vi "AI test.vi"() -> ()   [LabVIEW 2017]
panel:
  in  "Reade":bool
  in  "stop":bool
  out "AI  Init  array":errorcluster[](array[cluster])
  out "Analog error":bool
  out "Analog Fault Counts":i32[](array[numeric])
  out "AI Data 0":waveform(dbl)[](graph)
  out "AI Data 1":waveform(dbl)[](graph)
  out "AI Data 2":waveform(dbl)[](graph)
  out "AI Error":errorcluster[](array[cluster])
  out "AI loop time":dbl format="%.6g"
  out "AI data 2":waveform(dbl)[](array[waveform])
  out "AI data 1":waveform(dbl)[](array[waveform])
  out "AI data 0":waveform(dbl)[](array[waveform])
  in  "RATE (Hz)":dbl=5000.0
  out "physical channels 2":string="DemoDevice,BID#0/ai0:1" caption="property value"
  out "physical channels 1":string="DemoDevice,BID#0/ai0:1" caption="property value"
  out "physical channels 0":string="DemoDevice,BID#0/ai0:1" caption="property value"
  out "AI Task2":u32
  out "AI Task1":u32
  out "AI Task0":u64
  in  "SAMPLES":dbl=500.0
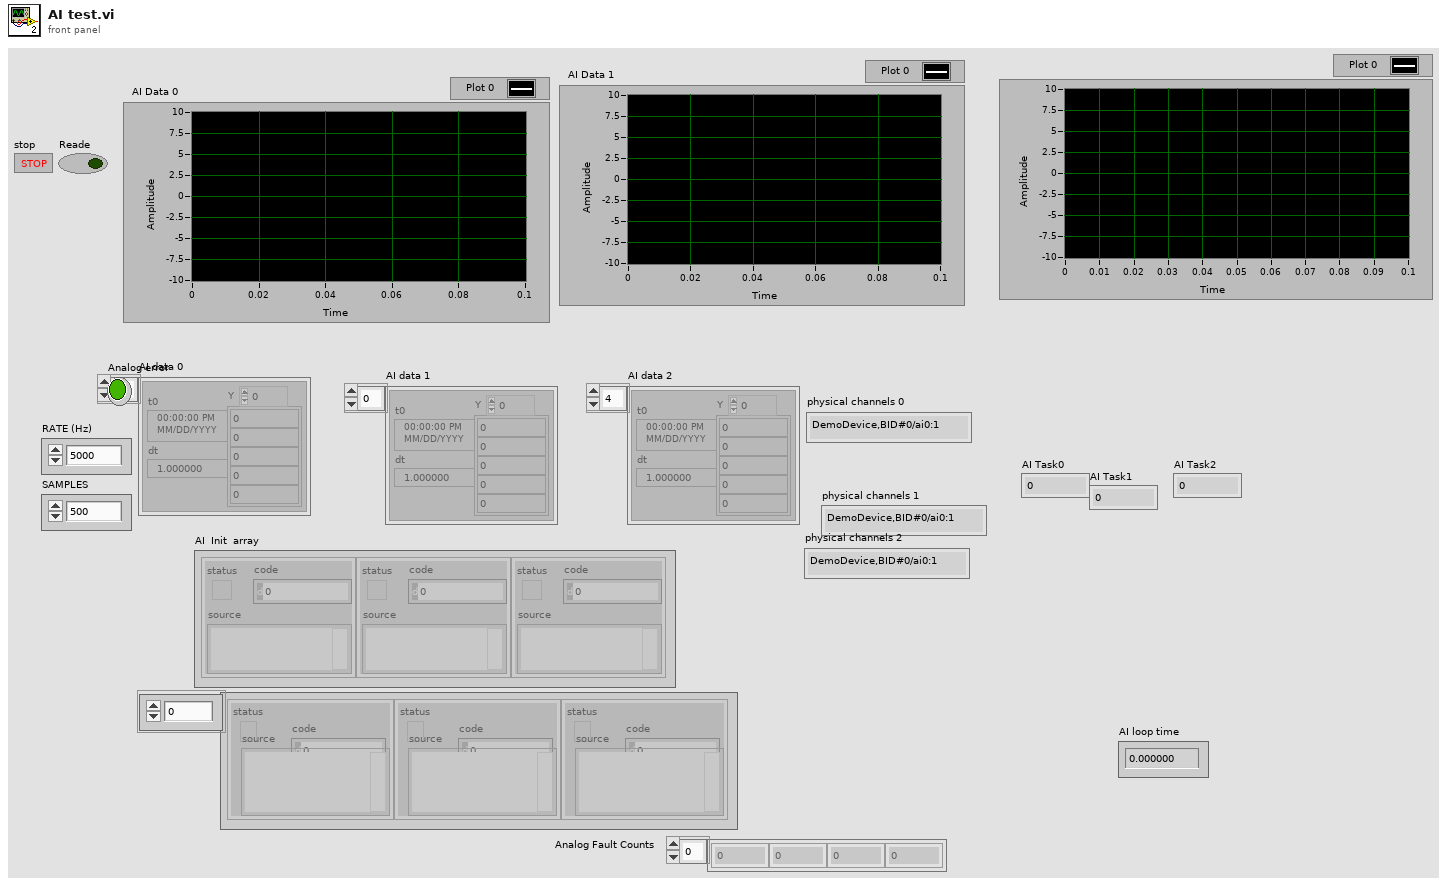
[diagram p1: front panel]
types:
  T1 = cluster{"OUT SERVER ADDRESS":string, "FROM ACCOUNT":string, "USER NAME":string, "PASSWORD":string, "TEST MAIL":bool, "TEST MAIL STATUS":string, "mail error":errorcluster}
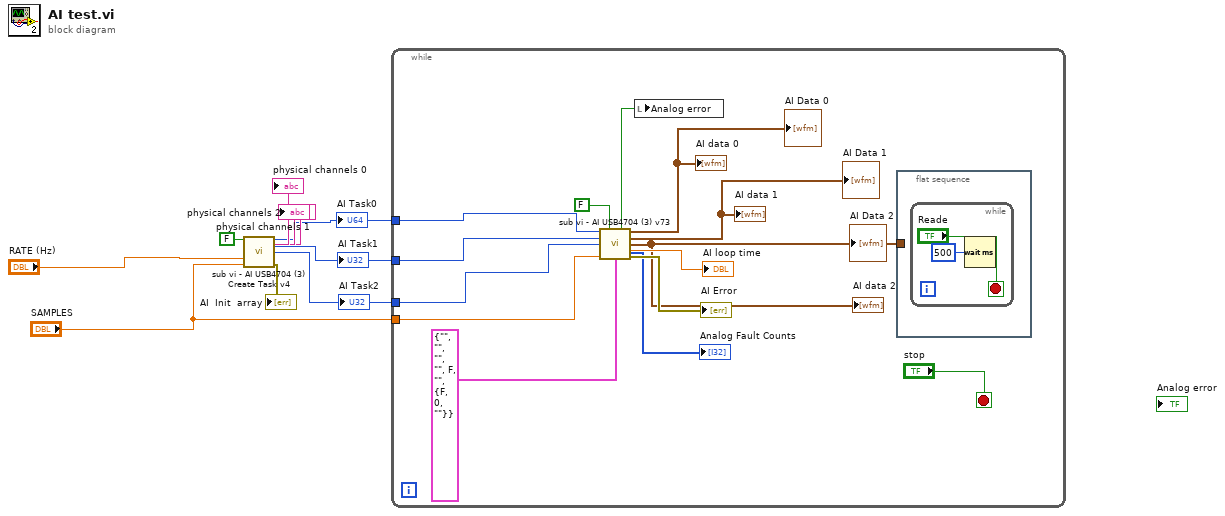
[diagram p0: block diagram]
diagram:
  n1 = call "sub vi - AI USB4704 (3)  Create Task v4.vi"("Test"=FALSE, "Rate Hz"="RATE (Hz)", "Samples"="SAMPLES") -> ("physical channels 0"=→"physical channels 0":string, "physical channels 1"=→"physical channels 1":string, "physical channels 2"=→"physical channels 2":string, "TASK USB 0"=w6:i32, "TASK USB 1"=w5:i32, "TASK USB 2"=w4:i32, "error array"=→"AI  Init  array":errorcluster[])  [unwired: 5 in, 1 out]
  "AI Task0" <- w6
  "AI Task1" <- w5
  "AI Task2" <- w4
  n2 = while {
    tunnel: w6 -> [w18]
    tunnel: w5 -> [w17]
    tunnel: w4 -> [w16]
    tunnel: "SAMPLES" -> [w14]
    stop <- "stop" stop-if-true
    n3 = call "sub vi - AI USB4704 (3) v73.vi"("Task0"=w18, "Test"=FALSE, "Task1"=w17, "Task2"=w16, "SAMPLES"=w14, "MAIL SETTINGS"=T1 {"OUT SERVER ADDRESS"="", "FROM ACCOUNT"="", "USER NAME"="", "PASSWORD"="", "TEST MAIL"=FALSE, "TEST MAIL STATUS"="", "mail error"={"status"=FALSE, "code"=0, "source"=""}}) -> ("Fault"=w19:bool, "data 0"=→"AI data 0" →"AI Data 0":waveform(dbl)[], "data 1"=→"AI data 1" →"AI Data 1":waveform(dbl)[], "data 2"=w13:waveform(dbl)[], "loop time"=→"AI loop time":dbl, "Fault Counts"=→"Analog Fault Counts":i32[], "error array"=→"AI Error":errorcluster[])  [unwired: 3 in]
    "AI data 2" <- w13
    "AI Data 2" <- w13
    n4 = local write "Analog error"(w19) -> ()
    n5 = flat-sequence {
      tunnel: w13 -> [_]
      frame #0 {
        n6 = while {
          stop <- "Reade" stop-if-true
          n7 = Wait (ms)(milliseconds to wait=u32 500) -> ()  [unwired: 1 out]
        }
      }
    }
  }
